vi "Convert Coordinates Array to Vertices.vi"(8 "Error In":errorcluster, 11 "Coordinates in":i32[](array[numeric])) -> (0 "Error Out":errorcluster, 3 "Vertices out":cluster{"X":dbl, "Y":dbl}[](array[cluster]))   [LabVIEW 2021, in "Image.lvlib"]
uses:
  Image.lvlib
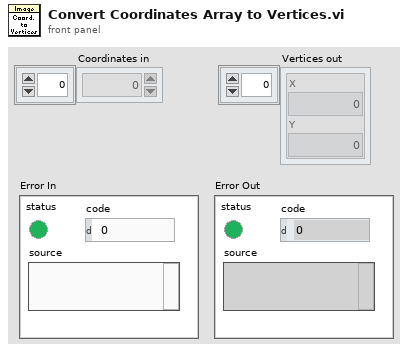
[diagram p1: front panel]
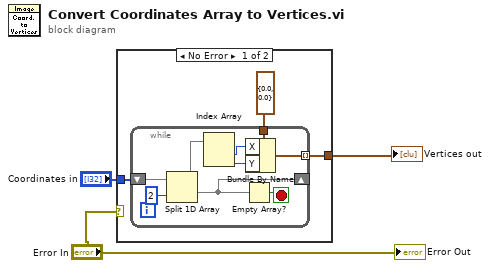
[diagram p0: block diagram]
diagram:
  n1 = case shown="No Error" "Error In" {
    tunnel: [w6 _] -> w3
    tunnel: "Coordinates in" -> [w4 _]
    frame No Error {
      n2 = while {
        shift-right: [w13] -> _
        shift-left: w4 -> [w15]
        tunnel: cluster{"X":dbl, "Y":dbl} {"X"=0.0, "Y"=0.0} ("Line End Points") -> [w11]
        tunnel: [w8] -> w6 mode=indexing
        stop <- w7 stop-if-true
        n3 = Split 1D Array(array=w15, index=2) -> (first subarray=w12:i32[], second subarray=w13:i32[])
        n4 = Index Array(array=w12) -> (element #1=w10:i32, element #2=w9:i32)  [unwired: 2 in]
        n5 = Empty Array?(array=w13) -> (empty?=w7:bool)
        n6 = Bundle By Name(cluster=w11, "X"=w10, "Y"=w9) -> (w8:cluster{"X":dbl, "Y":dbl})
      }
    }
    frame Error {
    }
  }
  "Vertices out" <- w3
  "Error Out" <- "Error In"
